vi "Areotech set enable.vi"(8 "error in (no error)":errorcluster, 10 "Parsed CMD":T1, 11 "AerotechStage in":refnum<class "AerotechStage.lvclass">) -> (0 "error out":errorcluster, 2 "new commands":string, 3 "AerotechStage out":refnum<class "AerotechStage.lvclass">)   [LabVIEW 2020, in "AerotechStage.lvclass"]
uses:
  AerotechStage.lvclass
  parsed device cmd.ctl
  OnOffTypeDef.ctl
  AerotechStage.lvclass/AerotechStage.ctl
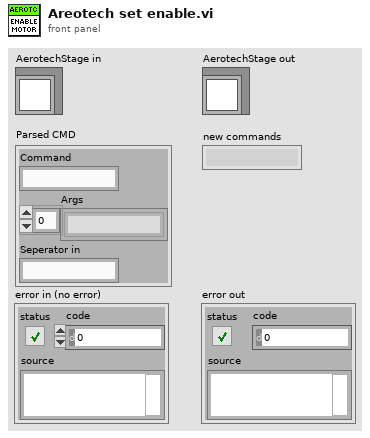
[diagram p1: front panel]
types:
  T1 = typedef "parsed device cmd.ctl" = cluster{"Command":string, "Args":string[], "Seperator in":string}
  T2 = typedef "OnOffTypeDef.ctl" = enum16{"off", "on"}
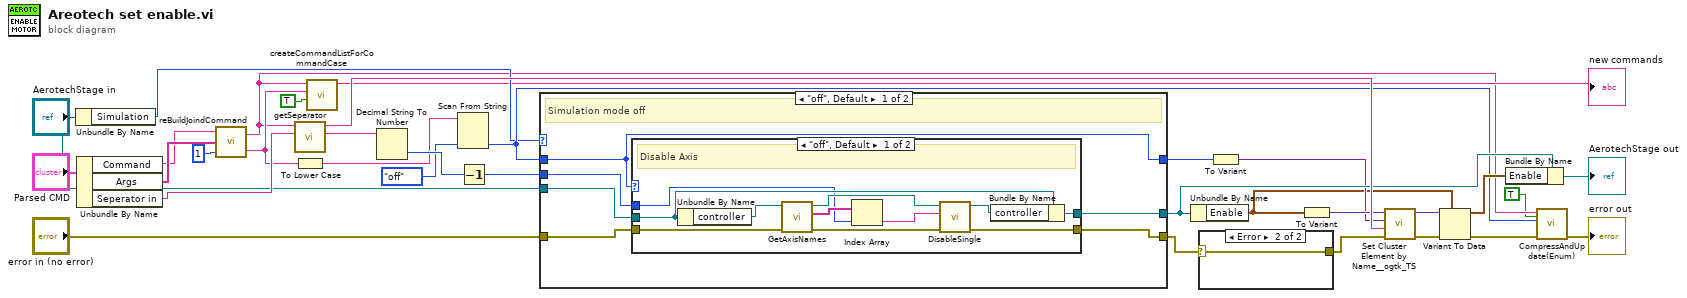
[diagram p0: block diagram]
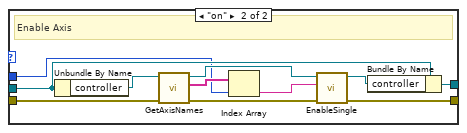
[diagram p3: hidden frame]
diagram:
  n1 = Unbundle By Name("AerotechStage in") -> ("Simulation"=w10:T2)
  n2 = Unbundle By Name("Parsed CMD") -> ("Command"=w31:string, "Args"=w32:string[], "Seperator in"=w33:string)
  n3 = call "reBuildJoindCommand.vi"("number of group elements (0)"=1, "Args"=w32, "Command 2"=w31) -> ("Arg"=w12:string, "Command"=w6:string)
  n4 = call "getSeperator.vi"("Channel Seperator (\"\")"=w33, "Command"=w6) -> ("Channel"=w18:string, "Seperator (e.g. \"Channel1\")"=w29:string)  [unwired: 8 in]
  n5 = To Lower Case(string=w12) -> (all lower case string=w11:string)
  n6 = call "createCommandListForCommandCase.vi"("immediate Check (only once)"=TRUE, "setvalue"=w12, "command"=w6) -> ("new commands"=→"new commands":string)  [unwired: 8 in]
  n7 = Decimal String To Number(string=w18) -> (number=w16:i32)  [unwired: 2 in, 1 out]
  n8 = Scan From String(input string=w11, default 1=OnOffTypeDef."off" ("Settings.Enable.Axis 1")) -> (output 1=w14:T2)  [unwired: 3 in, 3 out]
  n9 = Decrement(x=w16) -> (x-1=w17:i32)
  n10 = case shown="\"off\", Default" w10 {
    tunnel: "AerotechStage in" -> [w39 w64]
    tunnel: "error in (no error)" -> [w37 w63]
    tunnel: [w36 w63] -> w2
    tunnel: [w38 w64] -> w25
    tunnel: w14 -> [w34 w62]
    tunnel: w17 -> [w35 _]
    tunnel: [w34 w62] -> w27
    frame "off", Default {
      # "Simulation mode off"
      n11 = case shown="\"off\", Default" w34 {
        tunnel: w39 -> [w48 w61]
        tunnel: [w47 w60] -> w38
        tunnel: w37 -> [w46 w53]
        tunnel: [w43 w58] -> w36
        tunnel: w35 -> [w40 w54]
        frame "off", Default {
          # "Disable Axis"
          n12 = Unbundle By Name(w48) -> ("controller"=w50:refnum<k24>)
          n13 = call "GetAxisNames.vi"("error in (no error)"=w46, "controller in"=w50) -> ("error out"=w41:errorcluster, "axis names"=w49:string[], "controller out"=w45:refnum<k24>)  [unwired: 7 in]
          n14 = Index Array(array=w49, index=w40) -> (element=w44:string)
          n15 = call "DisableSingle.vi"("error in (no error)"=w41, "axis name"=w44, "controller in"=w45) -> ("error out"=w43:errorcluster, "controller out"=w42:refnum<k24>)  [unwired: 7 in]
          n16 = Bundle By Name(cluster=w48, "controller"=w42) -> (w47:refnum<class "AerotechStage.lvclass">)
        }
        frame "on" {
          # "Enable Axis"
          n17 = Unbundle By Name(w61) -> ("controller"=w57:refnum<k24>)
          n18 = call "GetAxisNames.vi"("error in (no error)"=w53, "controller in"=w57) -> ("error out"=w52:errorcluster, "axis names"=w55:string[], "controller out"=w56:refnum<k24>)  [unwired: 7 in]
          n19 = Index Array(array=w55, index=w54) -> (element=w51:string)
          n20 = call "EnableSingle.vi"("error in (no error)"=w52, "axis name"=w51, "controller in"=w56) -> ("error out"=w58:errorcluster, "controller out"=w59:refnum<k24>)  [unwired: 7 in]
          n21 = Bundle By Name(cluster=w61, "controller"=w59) -> (w60:refnum<class "AerotechStage.lvclass">)
        }
      }
    }
    frame "on" {
      # "Simulation mode on"
    }
  }
  n22 = Unbundle By Name(w25) -> ("Enable"=w21:cluster{"Axis1":T2, "Axis2":T2, "Axis3":T2})
  n23 = case shown="Error" w2 {
    selector: w2 -> [_ w65]
    tunnel: [_ w65] -> w1
    frame No Error {
    }
    frame Error {
    }
  }
  n24 = To Variant(anything=w27) -> (Variant=w23:variant)
  n25 = To Variant(anything=w21) -> (Variant=w24:variant)
  n26 = call "Set Cluster Element by Name__ogtk_TS.vi"("error in (no error)"=w1, "Element Name (\"\": New Element Data Name)"=w29, "New Element Value"=w23, "Cluster"=w24) -> ("error out"=w19:errorcluster, "VCluster out"=w20:variant)  [unwired: 5 in, 1 out]
  n27 = Variant To Data(error in=w19, type=w21, Variant=w20) -> (data=w22:cluster{"Axis1":T2, "Axis2":T2, "Axis3":T2}, error out=w28:errorcluster)
  n28 = Bundle By Name(cluster=w25, "Enable"=w22) -> (→"AerotechStage out":refnum<class "AerotechStage.lvclass">)
  n29 = call "CompressAndUpdate(Enum).vi"("force CVT update (false)"=TRUE, "error in"=w28, "enum variant"=w14, "command or variable name"=w6) -> ("error out"=→"error out":errorcluster)  [unwired: 7 in]
